vi "Get Strings from Ref.vi"(8 "error in (no error)":errorcluster, 9 "Label Prefix":string, 10 "GObj Refnum in":refnum<vi>, 11 "Decoration in":refnum<class "DecorationText.lvclass">) -> (0 "error out":errorcluster, 1 "Valid?":bool, 2 "GObj Refnum out":refnum<vi>, 3 "Decoration out":refnum<class "DecorationText.lvclass">, 4 "GObj Name":string)   [LabVIEW 2013, in "SET Project Data.lvlib" / "DecorationText.lvclass"]
uses:
  DecorationText.lvclass
  GObject/GObject.lvclass/GObject.ctl
  GObject/Write UID.vi
  GObject/Write ClassName.vi
  GObject/Write Label.vi
  GObject/GObject.lvclass
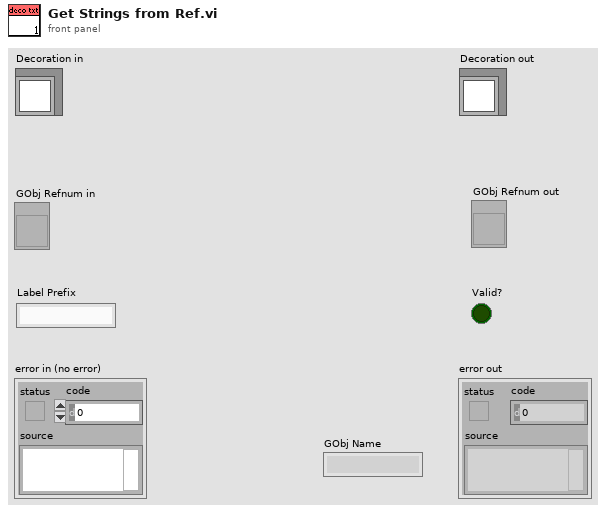
[diagram p1: front panel]
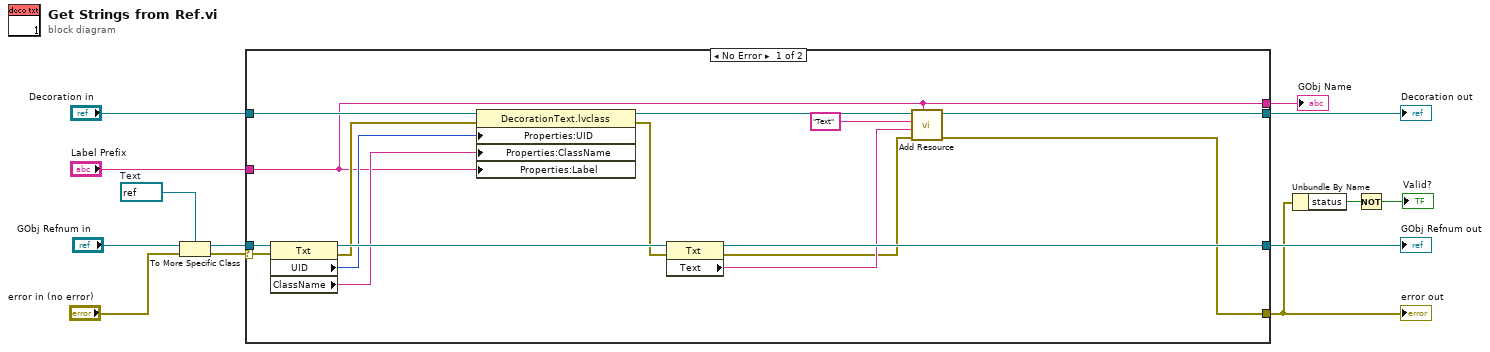
[diagram p0: block diagram]
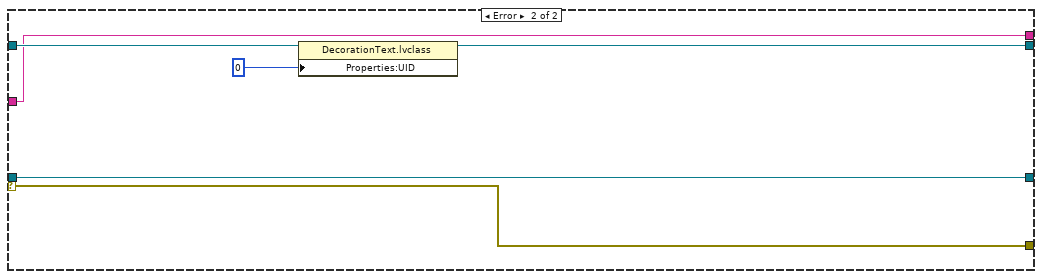
[diagram p2: hidden frame]
diagram:
  w7 = refnum<vi> refnum  # Text
  n1 = To More Specific Class(target class=w7, reference="GObj Refnum in", error in="error in (no error)") -> (specific class reference=w10:refnum<vi>, error out=w9:errorcluster)
  n2 = case shown="No Error" w9 {
    selector: w9 -> [w27 w35]
    tunnel: [w15 w35] -> w4
    tunnel: [w19 w32] -> w12
    tunnel: "Decoration in" -> [w26 w33]
    tunnel: w10 -> [w29 w34]
    tunnel: [w22 w34] -> w11
    tunnel: "Label Prefix" -> [w14 w30]
    tunnel: [w14 w30] -> w3
    frame No Error {
      n3 = property class="Txt"(reference=w29, error in=w27) -> (reference out=w28:refnum<vi>, error out=w24:errorcluster, "UID"=w21:i32, "ClassName"=w25:string)
      n4 = property class="DecorationText.lvclass"(reference=w26, error in=w24, "Properties:UID"=w21, "Properties:ClassName"=w25, "Properties:Label"=w14) -> (reference out=w20:refnum<class "DecorationText.lvclass">, error out=w23:errorcluster)
      n5 = property class="Txt"(reference=w28, error in=w23) -> (reference out=w22:refnum<vi>, error out=w16:errorcluster, "Text"=w18:string)
      n6 = call "Add Resource.vi"("TagPrefix"=w14, "error in (no error)"=w16, "ItemText"=w18, "ItemName"="Text", "GObject in"=w20) -> ("error out"=w15:errorcluster, "GObject out"=w19:refnum<class "DecorationText.lvclass">)  [unwired: 5 in]
    }
    frame Error {
      n7 = property class="DecorationText.lvclass"(reference=w33, "Properties:UID"=0 ("UID")) -> (reference out=w32:refnum<class "DecorationText.lvclass">)  [unwired: 1 in, 1 out]
    }
  }
  "error out" <- w4
  "Decoration out" <- w12
  "GObj Refnum out" <- w11
  "GObj Name" <- w3
  n8 = Unbundle By Name(w4) -> ("status"=w2:bool)
  n9 = Not(x=w2) -> (.not. x?=→"Valid?":bool)
